vi "VisualStim.vi"(4 "Stim Parameters":T1={"Samples"=800, "Fstim"=0.125, "Slope"=8.0, "Fsampling"=100.0, "Amplitude"=100.0} {"Slope" format="%#_13g"}) -> (0 "Vel":dbl[](array[numeric]), 1 "Waveform Graph":dbl[][](graph))   [LabVIEW 2013]
doc: "Generates a OKS given the stimuli parameters. Provides Position (P). Velocity (V), and Acceleration (A)"
uses:
  <vilib>/Analysis/NI_AALBase.lvlib
  <vilib>/Analysis/NI_AALPro.lvlib
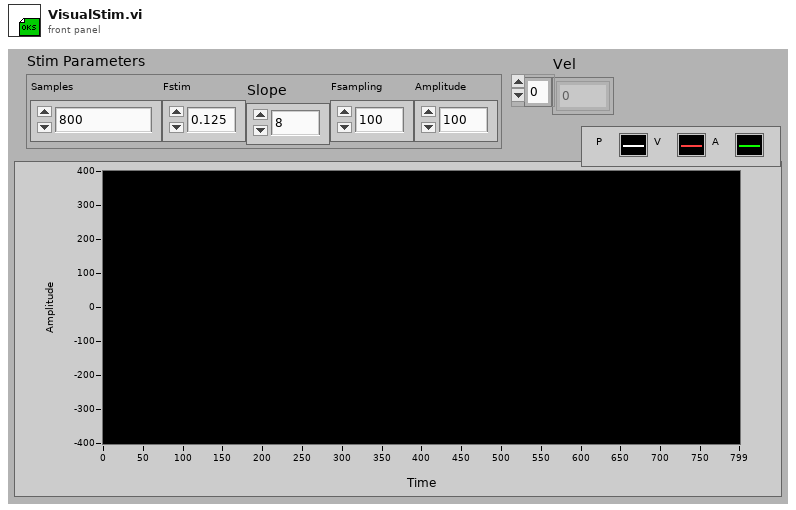
[diagram p1: front panel]
types:
  T1 = cluster{"Samples":i32, "Fstim":dbl, "Slope":dbl, "Fsampling":dbl, "Amplitude":dbl}
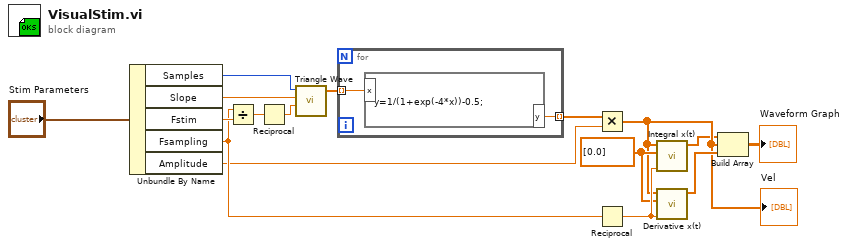
[diagram p0: block diagram]
diagram:
  w5 = dbl[] [0.0] ("Initial Condition")
  n1 = Unbundle By Name("Stim Parameters") -> ("Samples"=w10:i32, "Slope"=w9:dbl, "Fstim"=w8:dbl, "Fsampling"=w7:dbl, "Amplitude"=w3:dbl)
  n2 = Divide(x=w7, y=w8) -> (x/y=w16:dbl)
  n3 = Reciprocal(x=w16) -> (1/x=w15:dbl)
  n4 = call <vilib>:"Triangle Wave.vi"("samples"=w10, "amplitude"=w9, "frequency"=w15) -> ("triangle wave"=w14:dbl[])  [unwired: 2 in, 2 out]
  n5 = for {
    tunnel: [w18] -> w4 mode=indexing
    tunnel: w14 -> [w17] mode=indexing
    n6 = formula code="y=1/(1+exp(-4*x))-0.5;"("x"=w17) -> ("y"=w18:dbl)
  }
  n7 = Multiply(x=w4, y=w3) -> (x*y=w2:dbl[])
  "Vel" <- w2
  n8 = Reciprocal(x=w7) -> (1/x=w6:dbl)
  n9 = call <vilib>:"Integral x(t).vi"("dt"=w6, "Initial Condition"=w5, "X"=w2) -> ("Integral X"=w1:dbl[])  [unwired: 7 in, 1 out]
  n10 = call <vilib>:"Derivative x(t).vi"("dt"=w6, "Initial Condition"=w5, "X"=w2) -> ("dX/dt"=w12:dbl[])  [unwired: 7 in, 1 out]
  n11 = Build Array(w1, w2, w12) -> (→"Waveform Graph":dbl[][])
